vi "17-ySteps&VelocityToPosition.vi"(10 "vy":i32, 11 "n":i32) -> (3 "y":dbl)   [LabVIEW 2019, in "17.lvlib"]
uses:
  17.lvlib
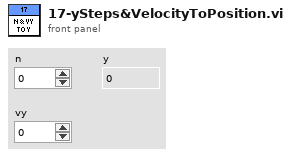
[diagram p1: front panel]
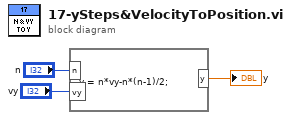
[diagram p0: block diagram]
diagram:
  n1 = formula code="y = n*vy-n*(n-1)/2;"("n"="n", "vy"="vy") -> ("y"=→"y":dbl)
